vi "Write Mass.vi"(10 "Mass":dbl, 11 "Movable in":refnum<class "Movable.lvclass">) -> (3 "Movable out":refnum<class "Movable.lvclass">)   [LabVIEW 2024, in "Movable.lvclass"]
doc: "MIT Licence\nCopyright (c) 2024 David Grollier"
uses:
  Movable.lvclass
  Movable.lvclass/Movable.ctl
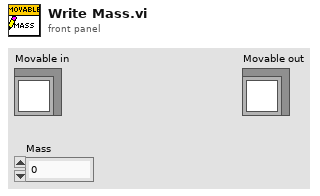
[diagram p1: front panel]
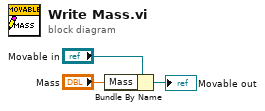
[diagram p0: block diagram]
diagram:
  n1 = Bundle By Name(cluster="Movable in", "Mass"="Mass") -> (→"Movable out":refnum<class "Movable.lvclass">)
